vi "Choreo_ByteBuffer_decode_Boolean.vi"(9 "StartByte":i32, 11 "RawData":u8[](array[numeric])) -> (1 "NextByte":i32, 3 "Boolean_Value":bool)   [LabVIEW 2019, in "ChoreoLib.lvlib"]
doc: "Decode (or strip out) a boolean from an array of bytes. No conversion or decoding is actually done, the memory is just copied, and the value is cast to the correct type. A TRUE boolean is stroed as an integer value = 1.\n\nInputs\n - RawData -- Array of bytes containing the data to be extracted.\n - StartByte -- The starting byte number (the first byte starts at 0)\n\nOutputs\n - Boolean_Value -- Boolean value.\n - NextByte -- The starting byte index for the next value (regardless of type)."
uses:
  ChoreoLib.lvlib
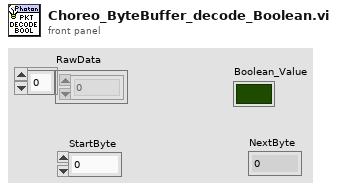
[diagram p1: front panel]
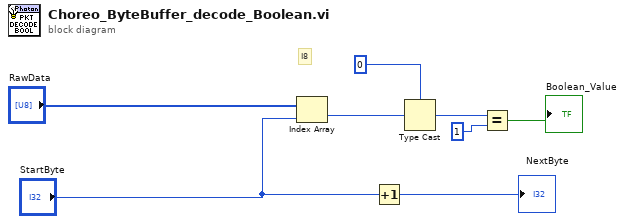
[diagram p0: block diagram]
diagram:
  # "I8"
  n1 = Index Array(array="RawData", index="StartByte") -> (element=w6:u8)
  n2 = Increment(x="StartByte") -> (x+1=→"NextByte":i32)
  n3 = Type Cast(type=i8 0, x=w6) -> (*(type *) &x=w3:i8)
  n4 = Equal?(x=w3, y=i8 1) -> (x = y?=→"Boolean_Value":bool)
